vi "Binary Stream.vi"() -> ()   [LabVIEW 2019]
uses:
  <vilib>/Instr/_visa.llb/VISA Configure Serial Port (Instr).vi
panel:
  in  "Value":dbl
  in  "CMD":u8(ring)=2 items=["Set Max"=2, "Set Min"=3]
  in  "Send":bool
  out "Chart":dbl(graph)
  out "error out":errorcluster
  in  "stop":bool
  in  "VISA resource name":refnum<visa-resource-name>
  # "Test this VI by first running Binary Streaming Instrument.vi.  You will need 2 serial ports that are connected via a NULL Modem cable."
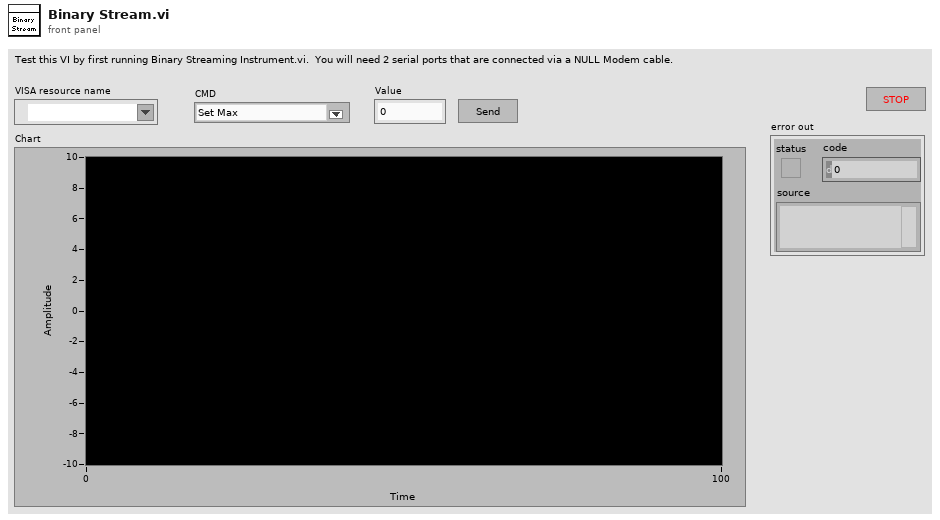
[diagram p1: front panel]
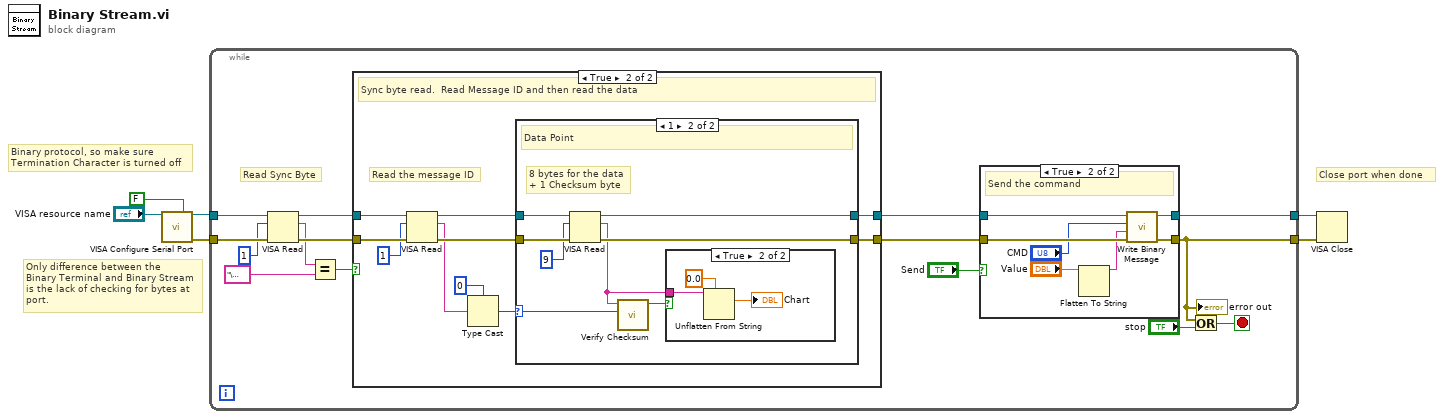
[diagram p0: block diagram]
diagram:
  # "Only difference between the\nBinary Terminal and Binary Stream\nis the lack of checking for bytes at\nport."
  # "Binary protocol, so make sure\nTermination Character is turned off"
  # "Close port when done"
  n1 = call-poly "VISA Configure Serial Port"("VISA resource name"="VISA resource name", "Enable Termination\nChar (T)"=FALSE ("Enable Termination\nChar (T)")) -> ("VISA resource name out"=w1:refnum<visa-resource-name>, "error out"=w5:errorcluster)  [unwired: 12 in]
  n2 = while {
    tunnel: w5 -> [w21]
    tunnel: w1 -> [w17]
    tunnel: [w16] -> w3
    tunnel: [w18] -> w6
    stop <- w15 stop-if-true
    # "Read Sync Byte"
    n3 = VISA Read(VISA resource name=w17, byte count=u32 1, error in (no error)=w21) -> (VISA resource name out=w11:refnum<visa-resource-name>, read buffer=w10:string, error out=w20:errorcluster)  [unwired: 1 out]
    n4 = Equal?(x=w10, y="\u0002") -> (x = y?=w8:bool)
    n5 = case shown="True" w8 {
      tunnel: w11 -> [w22 w29]
      tunnel: w20 -> [w23 w33]
      tunnel: [w22 w24] -> w7
      tunnel: [w23 w31] -> w19
      frame False {
        # "Sync byte was not read.  Ignore the data assuming we are in the middle of a message."
      }
      frame True {
        # "Read the message ID"
        # "Sync byte read.  Read Message ID and then read the data"
        n6 = VISA Read(VISA resource name=w29, byte count=u32 1, error in (no error)=w33) -> (VISA resource name out=w25:refnum<visa-resource-name>, read buffer=w28:string, error out=w32:errorcluster)  [unwired: 1 out]
        n7 = Type Cast(type=u8 0, x=w28) -> (*(type *) &x=w26:u8)
        n8 = case shown="1" w26 {
          selector: w26 -> [_ w37]
          tunnel: w32 -> [w35 w43]
          tunnel: w25 -> [w34 w41]
          tunnel: [w34 w39] -> w24
          tunnel: [w35 w42] -> w31
          frame Default {
            # "Unknown ID.  Ignore the data"
          }
          frame 1 {
            # "8 bytes for the data\n+ 1 Checksum byte"
            # "Data Point"
            n9 = VISA Read(VISA resource name=w41, byte count=u32 9, error in (no error)=w43) -> (VISA resource name out=w39:refnum<visa-resource-name>, read buffer=w36:string, error out=w42:errorcluster)  [unwired: 1 out]
            n10 = call "Verify Checksum.vi"("Message ID"=w37, "Data + Checksum"=w36) -> ("Pass"=w38:bool)  [unwired: 9 in]
            n11 = case shown="True" w38 {
              tunnel: w36 -> [_ w46]
              frame False {
              }
              frame True {
                n12 = Unflatten From String(type=0.0, binary string=w46) -> (value=→"Chart":dbl)  [unwired: 3 in, 2 out]
              }
            }
          }
        }
      }
    }
    n13 = case shown="True" "Send" {
      tunnel: [w48 w55] -> w18
      tunnel: [w47 w53] -> w16
      tunnel: w7 -> [w47 w52]
      tunnel: w19 -> [w48 w54]
      frame False {
        # "Do nothing"
      }
      frame True {
        # "Send the command"
        n14 = Flatten To String(anything="Value") -> (data string=w49:string)  [unwired: 3 in, 2 out]
        n15 = call "Write Binary Message.vi"("error in"=w54, "Flattened Data"=w49, "Message ID"="CMD", "VISA resource in"=w52) -> ("error out"=w55:errorcluster, "VISA resource out"=w53:refnum<visa-resource-name>)  [unwired: 6 in]
      }
    }
    "error out" <- w18
    n16 = Or(x=w18, y="stop") -> (x .or. y?=w15:bool)
  }
  n17 = VISA Close(VISA resource name=w3, error in (no error)=w6) -> ()  [unwired: 1 out]
